vi "Get LibItems from ProjectItem.vi"(8 "error in (no error)":errorcluster, 11 "ProjectItem in":refnum<vi>) -> (0 "error out":errorcluster, 1 "Library Item Names":string[](array[string]), 2 "Library Items":refnum<vi>[](array[refnum]), 3 "ProjectItem out":refnum<vi>)   [LabVIEW 2020, in "gRPC Scripting Tools.lvlib"]
uses:
  gRPC Scripting Tools.lvlib
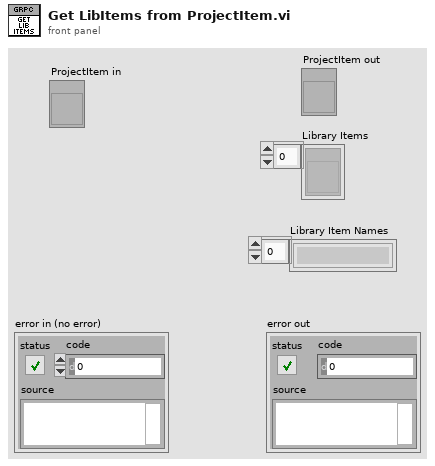
[diagram p1: front panel]
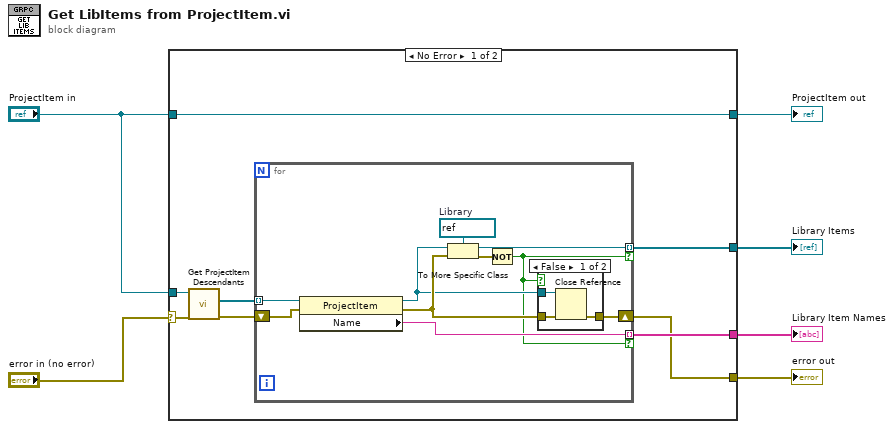
[diagram p0: block diagram]
diagram:
  n1 = case shown="No Error" "error in (no error)" {
    selector: "error in (no error)" -> [w7 w29]
    tunnel: "ProjectItem in" -> [w14 _]
    tunnel: [w12 _] -> w6
    tunnel: [w10 _] -> w1
    tunnel: [w9 w29] -> w5
    tunnel: "ProjectItem in" -> [w8 w30]
    tunnel: [w8 w30] -> w3
    frame No Error {
      n2 = call "Get ProjectItem Descendants.vi"("error in (no error)"=w7, "ProjectItem in"=w14) -> ("error out"=w13:errorcluster, "All Descendents"=w11:refnum<vi>[])  [unwired: 7 in, 1 out]
      n3 = for {
        tunnel: w11 -> [w24] mode=indexing
        tunnel: [w23] -> w12 mode=indexing if=w15
        tunnel: [w20] -> w10 mode=indexing if=w15
        shift-right: [w16] -> w9
        shift-left: w13 -> [w19]
        w22 = refnum<vi> refnum  # Library
        n4 = property class="ProjectItem"(reference=w24, error in=w19) -> (reference out=w17:refnum<vi>, error out=w18:errorcluster, "Name"=w23:string)
        n5 = To More Specific Class(target class=w22, reference=w17, error in=w18) -> (specific class reference=w20:refnum<vi>, error out=w21:errorcluster)
        n6 = Not(x=w21) -> (.not. x?=w15:bool)
        n7 = case shown="False" w15 {
          tunnel: w18 -> [w27 w28]
          tunnel: w17 -> [w26 _]
          tunnel: [w25 w28] -> w16
          frame False {
            n8 = Close Reference(reference=w26, error in (no error)=w27) -> (error out=w25:errorcluster)
          }
          frame True {
          }
        }
      }
    }
    frame Error {
    }
  }
  "Library Item Names" <- w6
  "ProjectItem out" <- w3
  "error out" <- w5
  "Library Items" <- w1
